vi "Is_Library_Type.vi"(8 "error in (no error)":errorcluster, 11 "AB_Source_Library in":refnum<class "AB_Source_Library.lvclass">) -> (0 "error out":errorcluster, 1 "LVLIBPtopLevel":bool, 2 "library type":bool, 3 "AB_Source_Library out":refnum<class "AB_Source_Library.lvclass">)   [LabVIEW 2020, in "AB_Source_Library.lvclass"]
uses:
  <vilib>/AppBuilder/AB_Classes/Source/Library/AB_Source_Library.lvclass
  <vilib>/AppBuilder/AB_Classes/Source/Library/AB_Source_Library.lvclass/AB_Source_Library.ctl
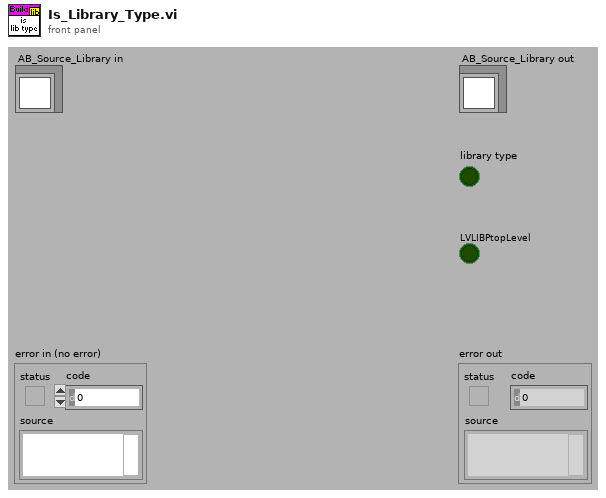
[diagram p1: front panel]
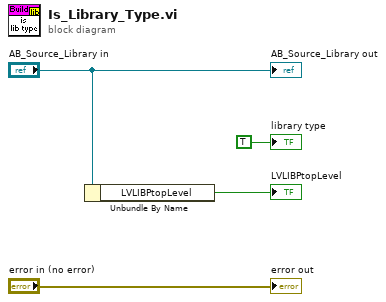
[diagram p0: block diagram]
diagram:
  n1 = Unbundle By Name("AB_Source_Library in") -> ("LVLIBPtopLevel"=→"LVLIBPtopLevel":bool)
  "error out" <- "error in (no error)"
  "AB_Source_Library out" <- "AB_Source_Library in"
  "library type" <- TRUE ("library type")
